vi "PH_SHS_Analysis_Statistician.add new result.vi"(0 "i ref in":refnum<vi>, 2 "SHS Analyzer Dataset":T1 {"State" items=["no info", "off/false/out", "on/true/in", "Failure", "Alarm", "Status 1", "Status 2", "Status 3"]; "Zernicke Coefficients"."2nd Spherical" scale=-2.0..2.0 scale format="%.2f"; "Zernicke Coefficients"."2nd Coma y" scale=-2.0..2.0 scale format="%.2f"; "Zernicke Coefficients"."2nd Coma x" scale=-2.0..2.0 scale format="%.2f"; "Zernicke Coefficients"."2nd Astig 45°" scale=-2.0..2.0 scale format="%.2f"; "Zernicke Coefficients"."2nd Astig 0°" scale=-2.0..2.0 scale format="%.2f"; "Zernicke Coefficients"."Trefoil 30°" scale=-2.0..2.0 scale format="%.2f"; "Zernicke Coefficients"."Trefoil 0°" scale=-2.0..2.0 scale format="%.2f"; "Zernicke Coefficients"."Spherical" scale=-2.0..2.0 scale format="%.2f"; "Zernicke Coefficients"."Coma y" scale=-2.0..2.0 scale format="%.2f"; "Zernicke Coefficients"."Coma x" scale=-2.0..2.0 scale format="%.2f"; "Zernicke Coefficients"."Astig 45°" scale=-2.0..2.0 scale format="%.2f"; "Zernicke Coefficients"."Astig 0°" scale=-2.0..2.0 scale format="%.2f"; "Zernicke Coefficients"."Defocus" scale=-2.0..2.0 scale format="%.2f"; "Zernicke Coefficients"."Tilt y" scale=-2.0..2.0 scale format="%.2f"; "Zernicke Coefficients"."Tilt x" scale=-2.0..2.0 scale format="%.2f"}, 5 "error in (no error)":errorcluster) -> (14 "i ref out":refnum<vi>, 19 "error out":errorcluster)   [LabVIEW 2014, in "PH_SHS_Analysis_Statistician.lvlib"]
doc: "This VI investigates the new incoming data and adds them to the results already collected."
uses:
  PH_SHS_Analysis_Statistician.lvlib
  PH_SHS_Analysis/PH_SHS_Analysis.Zernike Dataset.ctl
  PH_Basics/PH_StatusHandler/PH_StatusHandler.Status.ctl
  PH_SHS_Analysis/PH_SHS_Analysis.Zernike Coefficients.ctl
  PH_Basics/PH_Common/PH_Common.lvlib
  PH_SHS_Analysis/PH_SHS_Analysis.lvlib
  PH_Basics/PH_StatusHandler/PH_StatusHandler.lvlib
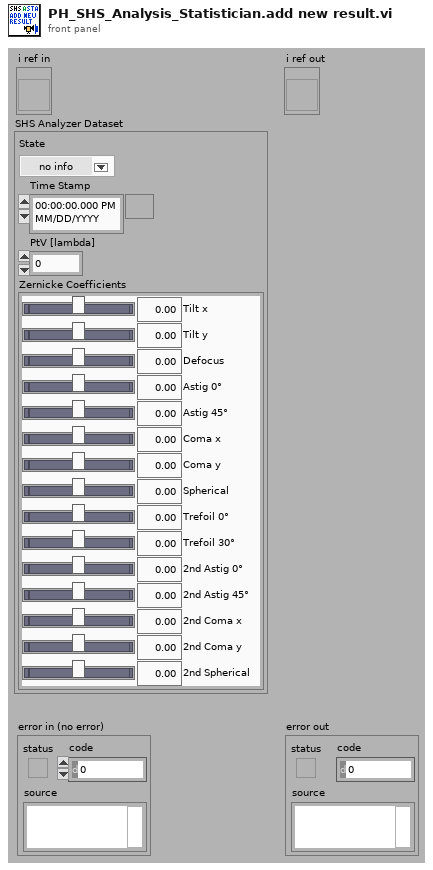
[diagram p1: front panel]
types:
  T1 = typedef "PH_SHS_Analysis.lvlib/PH_SHS_Analysis.Zernike Dataset.ctl" = cluster{"State":T2, "Time Stamp":timestamp, "PtV [lambda]":dbl, "Zernicke Coefficients":T3}
  T2 = typedef "PH_StatusHandler.lvlib/PH_StatusHandler.Status.ctl" = i16
  T3 = typedef "PH_SHS_Analysis.lvlib/PH_SHS_Analysis.Zernike Coefficients.ctl" = cluster{"Tilt x":dbl, "Tilt y":dbl, "Defocus":dbl, "Astig 0°":dbl, "Astig 45°":dbl, "Coma x":dbl, "Coma y":dbl, "Spherical":dbl, "Trefoil 0°":dbl, "Trefoil 30°":dbl, "2nd Astig 0°":dbl, "2nd Astig 45°":dbl, "2nd Coma x":dbl, "2nd Coma y":dbl, "2nd Spherical":dbl}
  T4 = typedef "PH_SHS_Analysis_Statistician.lvlib/PH_SHS_Analysis_Statistician.i attribute.ctl" = cluster{"GUI Refs ":cluster{"Status":refnum<vi>, "Result Graph":refnum<vi>, "Mean Data 1":refnum<vi>, "Std Dev Data 1":refnum<vi>, "Mean Data 2":refnum<vi>, "Std Dev Data 2":refnum<vi>, "Mean Data 3":refnum<vi>, "Std Dev Data 3":refnum<vi>, "Dummy Mean":refnum<vi>, "Dummy Std Dev":refnum<vi>, "Export Data":refnum<vi>, "Data 1":refnum<vi>, "Data 2":refnum<vi>, "Data 3":refnum<vi>, "Stat or Trend":refnum<vi>, "Delete":refnum<vi>, "Analyzer":refnum<vi>, "Current Zernike Coefficients":refnum<vi>, "PtV [Lambda]":refnum<vi>, "sample length":refnum<vi>}, "Analyzer":string, "Stat or Trend":bool, "Data 1":i16, "Data 2":i16, "Data 3":i16, "Data":T1[], "sample length":i32, "Datasets strored":i32, "Dataarray Size":i32}
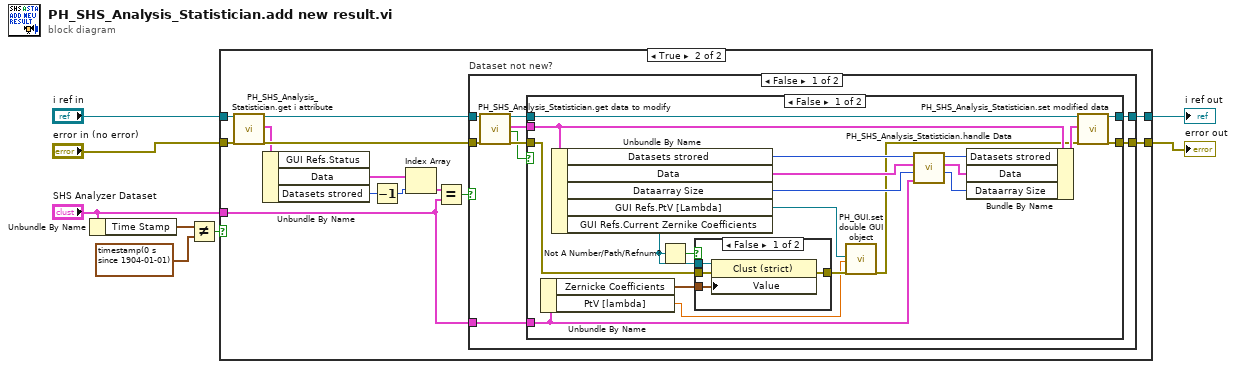
[diagram p0: block diagram]
diagram:
  n1 = Unbundle By Name("SHS Analyzer Dataset") -> ("Time Stamp"=w7:timestamp)
  n2 = Not Equal?(x=w7, y=timestamp(0 s since 1904-01-01)) -> (x != y?=w1:bool)
  n3 = case shown="True" w1 {
    tunnel: "SHS Analyzer Dataset" -> [_ w15]
    tunnel: [w9 w14] -> w5
    tunnel: [w10 w13] -> w4
    tunnel: "i ref in" -> [w10 w12]
    tunnel: "error in (no error)" -> [w9 w11]
    frame False {
    }
    frame True {
      n4 = call "PH_SHS_Analysis_Statistician.get i attribute.vi"("i ref in"=w12, "error in (no error)"=w11) -> ("i ref out"=w22:refnum<vi>, "i attribute"=w21:T4, "error out"=w23:errorcluster)  [unwired: 15 in]
      n5 = Unbundle By Name(w21) -> ("Data"=w18:T1[], "Datasets strored"=w16:i32)  [unwired: 1 out]
      n6 = Decrement(x=w16) -> (x-1=w19:i32)
      n7 = Index Array(array=w18, index=w19) -> (element=w20:T1)
      n8 = Equal?(x=w20, y=w15) -> (x = y?=w17:bool)
      n9 = case "Dataset not new?" shown="False" w17 {
        tunnel: [w29 w61] -> w13
        tunnel: w23 -> [w27 w60]
        tunnel: w22 -> [w26 w61]
        tunnel: [w25 w60] -> w14
        tunnel: w15 -> [w24 _]
        frame False {
          n10 = call "PH_SHS_Analysis_Statistician.get data to modify.vi"("i ref in"=w26, "error in (no error)"=w27) -> ("i ref out"=w30:refnum<vi>, "i attribute"=w32:T4, "timed out"=w28:bool, "error out"=w31:errorcluster)  [unwired: 14 in]
          n11 = case shown="False" w28 {
            tunnel: w32 -> [w46 _]
            tunnel: w31 -> [w37 w58]
            tunnel: [w52 w58] -> w25
            tunnel: w30 -> [w51 w59]
            tunnel: [w50 w59] -> w29
            tunnel: w24 -> [w38 _]
            frame False {
              n12 = Unbundle By Name(w38) -> ("Zernicke Coefficients"=w40:T3, "PtV [lambda]"=w33:dbl)
              n13 = Unbundle By Name(w46) -> ("Datasets strored"=w43:i32, "Data"=w42:T1[], "Dataarray Size"=w49:i32, "GUI Refs.PtV [Lambda]"=w34:refnum<vi>, "GUI Refs.Current Zernike Coefficients"=w35:refnum<vi>)
              n14 = Not A Number/Path/Refnum?(number/path/refnum=w35) -> (NaN/Path/Refnum?=w39:bool)
              n15 = case shown="False" w39 {
                tunnel: w37 -> [w56 w57]
                tunnel: [w55 w57] -> w41
                tunnel: w35 -> [w54 _]
                tunnel: w40 -> [w53 _]
                frame False {
                  n16 = property class="Clust (strict)"(reference=w54, error in=w56, "Value"=w53) -> (error out=w55:errorcluster)  [unwired: 1 out]
                }
                frame True {
                }
              }
              n17 = call "PH_GUI.set double GUI object.vi"("GUI object Ref"=w34, "value"=w33, "error in (no error)"=w41) -> ("error out"=w36:errorcluster)  [unwired: 16 in]
              n18 = call "PH_SHS_Analysis_Statistician.handle Data.vi"("New SHS Analyzer Dataset"=w38, "Dataarray Size in"=w49, "Data in"=w42, "Datasets strored in"=w43) -> ("Dataarray Size out"=w47:i32, "Data out"=w44:T1[], "Datasets strored out"=w45:i32)  [unwired: 3 in]
              n19 = Bundle By Name(cluster=w46, "Datasets strored"=w45, "Data"=w44, "Dataarray Size"=w47) -> (w48:T4)
              n20 = call "PH_SHS_Analysis_Statistician.set modified data.vi"("i ref in"=w51, "i attribute"=w48, "error in (no error)"=w36) -> ("i ref out"=w50:refnum<vi>, "error out"=w52:errorcluster)  [unwired: 15 in]
            }
            frame True {
            }
          }
        }
        frame True {
        }
      }
    }
  }
  "error out" <- w5
  "i ref out" <- w4
